vi "Get Aviable Memory.vi"(10 "error in (no error)":errorcluster, 11 "DataLength":i32) -> (2 "error out":errorcluster, 3 "MDPtr DVR":refnum<data-value>)   [LabVIEW 2017, in "MDPtr.lvlib" / "MDPtrMgr.lvclass"]
uses:
  MDPtrMgr.lvclass
  MDPtr TypeDef/MDPtr DataFrame-Memory.ctl
  MDPtr TypeDef/MDPtr DataFrame-Common.ctl
  <vilib>/Utility/Data Type/Type Definitions/Data Type.ctl
  <vilib>/Utility/Data Type/NI_Data Type.lvlib
  MDPtr.lvlib
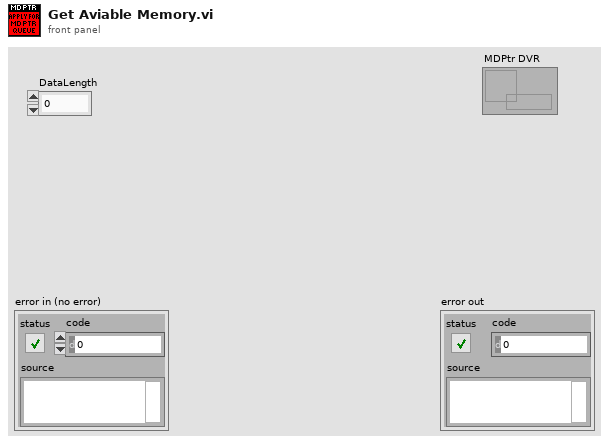
[diagram p1: front panel]
types:
  T1 = typedef "MDPtr.lvlib/MDPtr Queue.ctl" = refnum<queue>
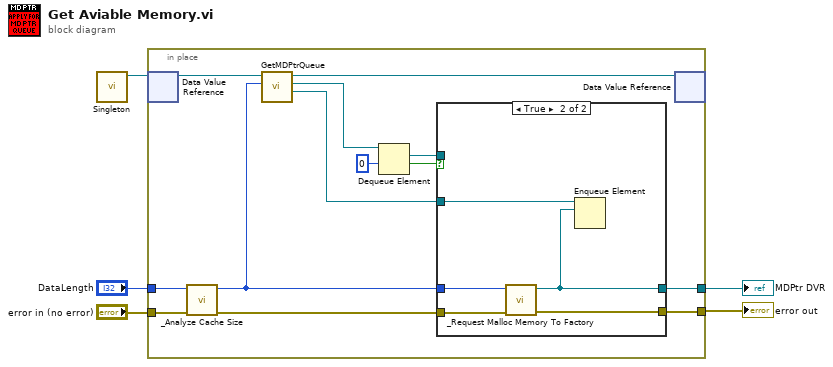
[diagram p0: block diagram]
diagram:
  n1 = call "Singleton.vi"() -> ("MDPtrMgrDVR"=w5:refnum<data-value>)  [unwired: 9 in, 2 out]
  n2 = in-place {
    in-place-border: "DataLength" -> [w7]
    in-place-border: [w13] -> w3
    in-place-border: [w12] -> w2
    in-place-border: "error in (no error)" -> [w9]
    n3 = in-place-dvr #1(w5) -> (w18:refnum<class "MDPtrMgr.lvclass">)  [unwired: 1 out]
    n4 = call "_Analyze Cache Size.vi"("error in (no error)"=w9, "DataSize"=w7) -> ("error out"=w8:errorcluster, "CacheSize"=w6:i32)  [unwired: 8 in]
    n5 = call "GetMDPtrQueue.vi"("CacheSize"=w6, "MDPtrMgr in"=w18) -> ("Total MDPtrQueue"=w10:T1, "MDPtrQueue"=w11:T1, "MDPtrMgr out"=w17:refnum<class "MDPtrMgr.lvclass">)  [unwired: 6 in, 1 out]
    n6 = Dequeue Element(queue=w11, timeout in ms (-1)=0) -> (element=w16:refnum<data-value>, timed out?=w15:bool)  [unwired: 1 in, 2 out]
    n7 = case shown="True" w15 {
      tunnel: [w19 w25] -> w13
      tunnel: w6 -> [_ w24]
      tunnel: [w20 w22] -> w12
      tunnel: w16 -> [w20 _]
      tunnel: w10 -> [_ w23]
      tunnel: w8 -> [w19 w21]
      frame False {
      }
      frame True {
        n8 = call "_Request Malloc Memory To Factory.vi"("error in (no error)"=w21, "CacheSize"=w24) -> ("error out"=w25:errorcluster, "MDPtr DVR"=w22:refnum<data-value>)  [unwired: 8 in]
        n9 = Enqueue Element(queue=w23, element=w22) -> ()  [unwired: 2 in, 3 out]
      }
    }
    n10 = in-place-dvr #1(w17) -> ()  [unwired: 2 out]
  }
  "error out" <- w3
  "MDPtr DVR" <- w2
